vi "Configure Dialog.vi"(8 "error in (no error)":errorcluster, 11 "Initiate Generation Msg in":refnum<class "Initiate Generation Msg.lvclass">) -> (0 "error out":errorcluster, 2 "Ok?":bool, 3 "Initiate Generation Msg out":refnum<class "Initiate Generation Msg.lvclass">)   [LabVIEW 2014, in "CS++Fgen.lvlib" / "Initiate Generation Msg.lvclass"]
uses:
  Initiate Generation Msg.lvclass
  Initiate Generation Msg.lvclass/Initiate Generation Msg.ctl
panel:
  in  "Initiate?":bool
  in  "OK Button":bool
  in  "Cancel Button":bool
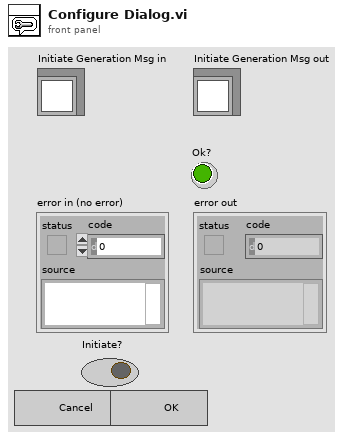
[diagram p1: front panel]
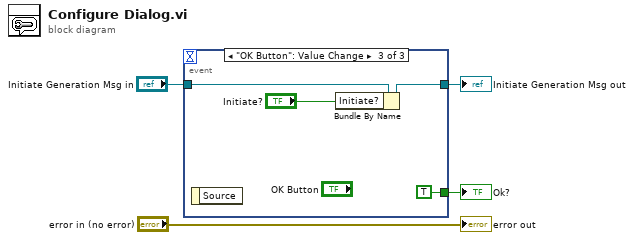
[diagram p0: block diagram]
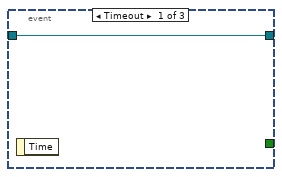
[diagram p2: hidden frame]
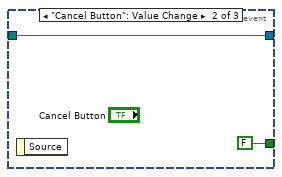
[diagram p3: hidden frame]
diagram:
  n1 = event shown="[2] \"OK Button\": Value Change" {
    selector: _ -> [_ _ _]
    dyn-events: _ -> [_ _ _]
    timeout: _ -> [_ _ _]
    tunnel: [w5 w7 w9] -> w3
    tunnel: "Initiate Generation Msg in" -> [w5 w7 w10]
    tunnel: [_ FALSE TRUE] -> w1
    event Timeout {
      n2 = event-data() -> ()  [unwired: 1 in, 1 out]
    }
    event "Cancel Button": Value Change {
      n3 = event-data() -> ()  [unwired: 1 in, 1 out]
    }
    event "OK Button": Value Change {
      n4 = event-data() -> ()  [unwired: 1 in, 1 out]
      n5 = Bundle By Name(cluster=w10, "Initiate?"="Initiate?") -> (w9:refnum<class "Initiate Generation Msg.lvclass">)
    }
  }
  "Initiate Generation Msg out" <- w3
  "Ok?" <- w1
  "error out" <- "error in (no error)"
